vi "Read Data Word Format.vi"(8 "error in (no error)":errorcluster, 11 "CSV Word Logger in":refnum<class "CSV Word Logger.lvclass">) -> (0 "error out":errorcluster, 2 "Data Word Format":T1, 3 "CSV Word Logger out":refnum<class "CSV Word Logger.lvclass">)   [LabVIEW 2023, in "Ballard MIL-STD-1553 Engine Support.lvlib" / "Implementation.lvlib" / "CSV Word Logger.lvclass"]
uses:
  CSV Word Logger.lvclass
  Shared/Data Word Format.ctl
  CSV Word Logger.lvclass/CSV Word Logger.ctl
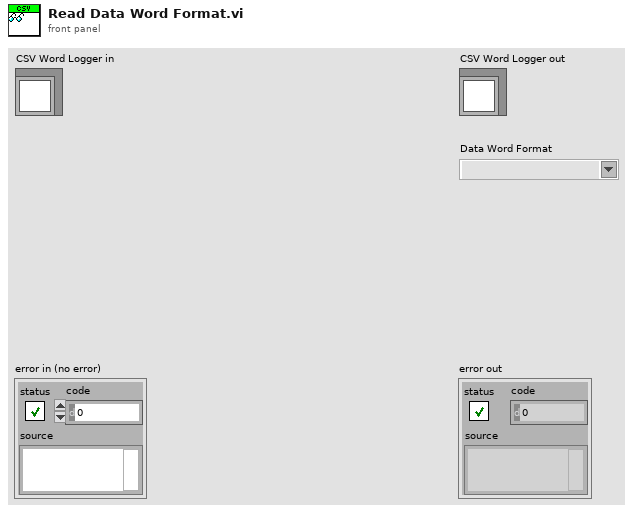
[diagram p1: front panel]
types:
  T1 = typedef "Data Word Format.ctl" = string
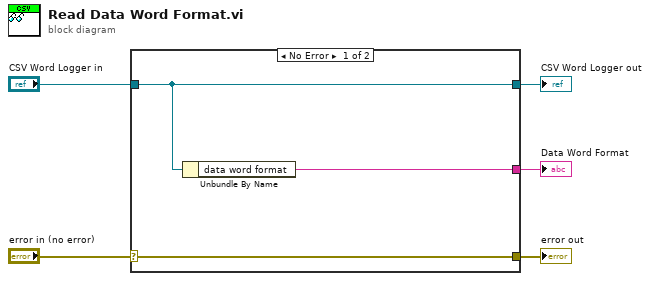
[diagram p0: block diagram]
diagram:
  n1 = case shown="No Error" "error in (no error)" {
    selector: "error in (no error)" -> [w8 w9]
    tunnel: [w8 w9] -> w4
    tunnel: [w7 w10] -> w2
    tunnel: "CSV Word Logger in" -> [w7 w10]
    tunnel: [w6 _] -> w1
    frame No Error {
      n2 = Unbundle By Name(w7) -> ("data word format"=w6:T1)
    }
    frame Error {
    }
  }
  "error out" <- w4
  "CSV Word Logger out" <- w2
  "Data Word Format" <- w1
